vi "obliczanie wzmocnienia.vi"() -> ()   [LabVIEW 2014]
uses:
  Obliczanie wzmocnienia Global.vi
panel:
  out "element":dbl
  out "Waveform z pelny":dbl[][](graph)
  out "Waveform z podzialem":dbl[][](graph)
  out "Waveform Uproszczony":dbl[][](graph)
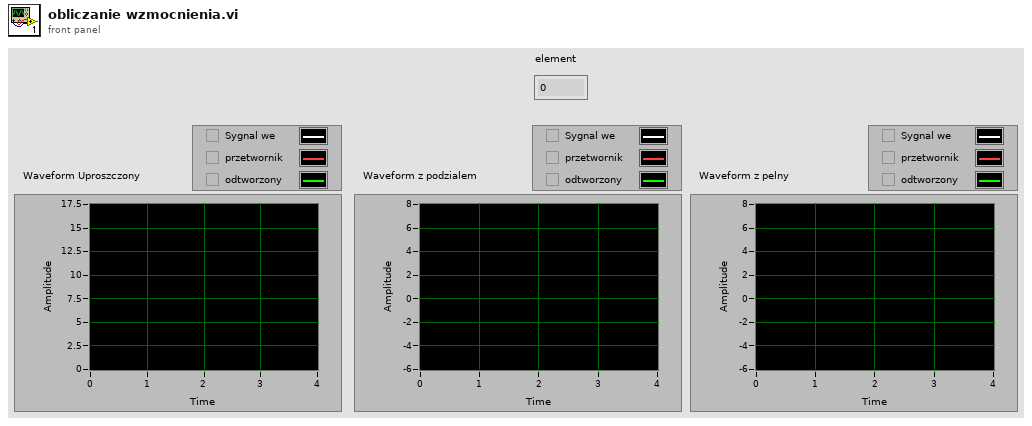
[diagram p1: front panel]
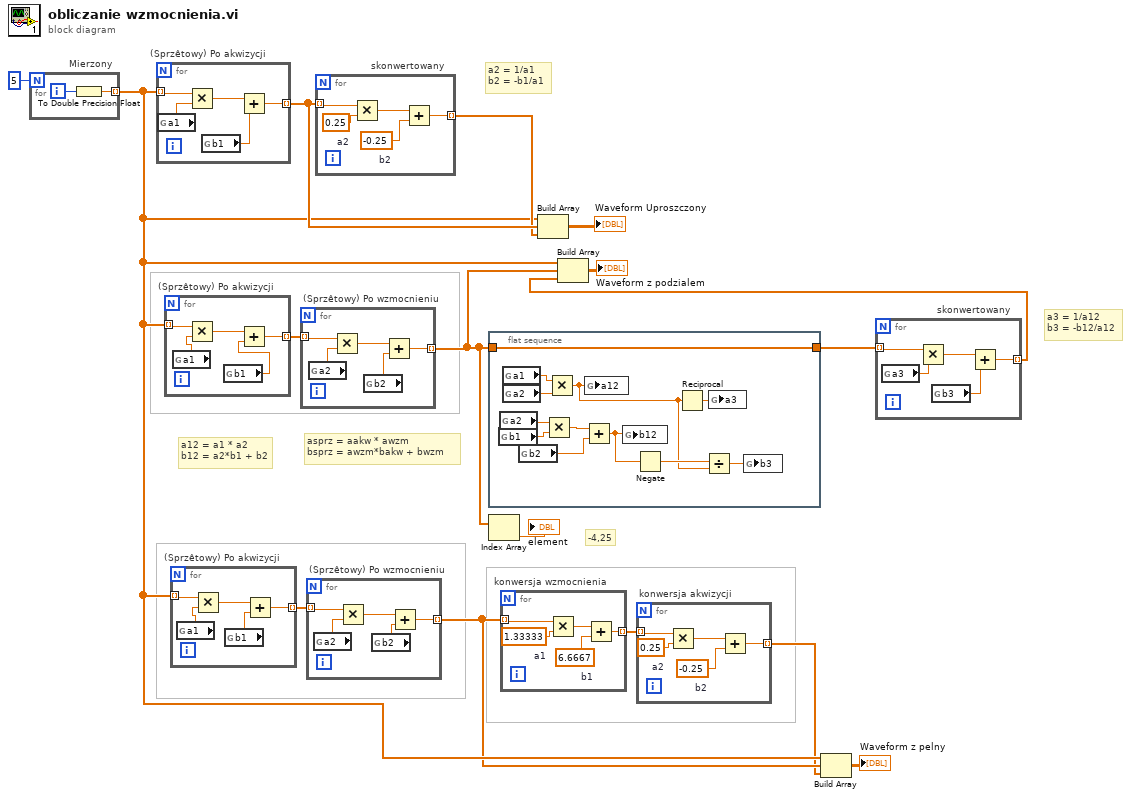
[diagram p0: block diagram]
diagram:
  # "asprz = aakw * awzm\nbsprz = awzm*bakw + bwzm"
  # "-4,25"
  # "a3 = 1/a12\nb3 = -b12/a12"
  # "a12 = a1 * a2\nb12 = a2*b1 + b2"
  # "a2 = 1/a1\nb2 = -b1/a1"
  n1 = for "Mierzony" {
    N: 5 -> [_]
    tunnel: [w17] -> w6 mode=indexing
    i -> [w18]
    n2 = To Double Precision Float(number=w18) -> (double precision float=w17:dbl)
  }
  n3 = for "(Sprzêtowy) Po akwizycji" {
    tunnel: w6 -> [w23] mode=indexing
    tunnel: [w21] -> w14 mode=indexing
    n4 = global read "Obliczanie wzmocnienia Global.vi" "a1"() -> (w20:dbl)
    n5 = Multiply(x=w23, y=w20) -> (x*y=w22:dbl)
    n6 = global read "Obliczanie wzmocnienia Global.vi" "b1"() -> (w19:dbl)
    n7 = Add(x=w22, y=w19) -> (x+y=w21:dbl)
  }
  n8 = for "(Sprzêtowy) Po akwizycji" {
    tunnel: w6 -> [w28] mode=indexing
    tunnel: [w26] -> w11 mode=indexing
    n9 = global read "Obliczanie wzmocnienia Global.vi" "a1"() -> (w25:dbl)
    n10 = Multiply(x=w28, y=w25) -> (x*y=w27:dbl)
    n11 = global read "Obliczanie wzmocnienia Global.vi" "b1"() -> (w24:dbl)
    n12 = Add(x=w27, y=w24) -> (x+y=w26:dbl)
  }
  n13 = for "(Sprzêtowy) Po akwizycji" {
    tunnel: w6 -> [w33] mode=indexing
    tunnel: [w31] -> w9 mode=indexing
    n14 = global read "Obliczanie wzmocnienia Global.vi" "a1"() -> (w30:dbl)
    n15 = Multiply(x=w33, y=w30) -> (x*y=w32:dbl)
    n16 = global read "Obliczanie wzmocnienia Global.vi" "b1"() -> (w29:dbl)
    n17 = Add(x=w32, y=w29) -> (x+y=w31:dbl)
  }
  n18 = for "(Sprzêtowy) Po wzmocnieniu" {
    tunnel: w11 -> [w38] mode=indexing
    tunnel: [w36] -> w3 mode=indexing
    n19 = global read "Obliczanie wzmocnienia Global.vi" "a2"() -> (w35:dbl)
    n20 = Multiply(x=w38, y=w35) -> (x*y=w37:dbl)
    n21 = global read "Obliczanie wzmocnienia Global.vi" "b2"() -> (w34:dbl)
    n22 = Add(x=w37, y=w34) -> (x+y=w36:dbl)
  }
  n23 = for "(Sprzêtowy) Po wzmocnieniu" {
    tunnel: w9 -> [w43] mode=indexing
    tunnel: [w41] -> w5 mode=indexing
    n24 = global read "Obliczanie wzmocnienia Global.vi" "a2"() -> (w40:dbl)
    n25 = Multiply(x=w43, y=w40) -> (x*y=w42:dbl)
    n26 = global read "Obliczanie wzmocnienia Global.vi" "b2"() -> (w39:dbl)
    n27 = Add(x=w42, y=w39) -> (x+y=w41:dbl)
  }
  n28 = for "skonwertowany" {
    tunnel: w14 -> [w48] mode=indexing
    tunnel: [w44] -> w13 mode=indexing
    w45 = -0.25  # b2
    w47 = 0.25  # a2
    n29 = Multiply(x=w48, y=w47) -> (x*y=w46:dbl)
    n30 = Add(x=w46, y=w45) -> (x+y=w44:dbl)
  }
  n31 = flat-sequence {
    tunnel: w3 -> [w49]
    tunnel: [w49] -> w1
    frame #0 {
      n32 = global read "Obliczanie wzmocnienia Global.vi" "b1"() -> (w56:dbl)
      n33 = global read "Obliczanie wzmocnienia Global.vi" "a2"() -> (w57:dbl)
      n34 = global read "Obliczanie wzmocnienia Global.vi" "a1"() -> (w59:dbl)
      n35 = global read "Obliczanie wzmocnienia Global.vi" "a2"() -> (w60:dbl)
      n36 = global read "Obliczanie wzmocnienia Global.vi" "b2"() -> (w54:dbl)
      n37 = Multiply(x=w57, y=w56) -> (x*y=w55:dbl)
      n38 = Multiply(x=w59, y=w60) -> (x*y=w51:dbl)
      n39 = Add(x=w55, y=w54) -> (x+y=w53:dbl)
      n40 = global write "Obliczanie wzmocnienia Global.vi" "a12"(w51) -> ()
      n41 = global write "Obliczanie wzmocnienia Global.vi" "b12"(w53) -> ()
      n42 = Negate(x=w53) -> (-x=w52:dbl)
      n43 = Reciprocal(x=w51) -> (1/x=w58:dbl)
      n44 = Divide(x=w52, y=w51) -> (x/y=w50:dbl)
      n45 = global write "Obliczanie wzmocnienia Global.vi" "a3"(w58) -> ()
      n46 = global write "Obliczanie wzmocnienia Global.vi" "b3"(w50) -> ()
    }
  }
  n47 = Index Array(array=w3) -> (element=→"element":dbl)  [unwired: 1 in]
  n48 = for "konwersja wzmocnienia" {
    tunnel: w5 -> [w65] mode=indexing
    tunnel: [w61] -> w8 mode=indexing
    w62 = 6.6667  # b1
    w64 = 1.33333  # a1
    n49 = Multiply(x=w65, y=w64) -> (x*y=w63:dbl)
    n50 = Add(x=w63, y=w62) -> (x+y=w61:dbl)
  }
  n51 = Build Array(w6, w14, w13) -> (→"Waveform Uproszczony":dbl[][])
  n52 = for "konwersja akwizycji" {
    tunnel: w8 -> [w70] mode=indexing
    tunnel: [w66] -> w4 mode=indexing
    w67 = -0.25  # b2
    w69 = 0.25  # a2
    n53 = Multiply(x=w70, y=w69) -> (x*y=w68:dbl)
    n54 = Add(x=w68, y=w67) -> (x+y=w66:dbl)
  }
  n55 = Build Array(w6, w5, w4) -> (→"Waveform z pelny":dbl[][])
  n56 = for "skonwertowany" {
    tunnel: w1 -> [w75] mode=indexing
    tunnel: [w73] -> w10 mode=indexing
    n57 = global read "Obliczanie wzmocnienia Global.vi" "a3"() -> (w72:dbl)
    n58 = Multiply(x=w75, y=w72) -> (x*y=w74:dbl)
    n59 = global read "Obliczanie wzmocnienia Global.vi" "b3"() -> (w71:dbl)
    n60 = Add(x=w74, y=w71) -> (x+y=w73:dbl)
  }
  n61 = Build Array(w6, w3, w10) -> (→"Waveform z podzialem":dbl[][])
